vi "LEBITlib.deviceToLoad.vi"(1 "DeviceName":string) -> (0 "DeviceIsToLoad":bool)   [LabVIEW 2014, in "LEBITLib.lvlib"]
doc: "Checks, if a device object must be instantiated. The following convention is used.\n\nIf the object name starts with a \"*\", the device object is ignored and will not be used"
uses:
  LEBITLib.lvlib
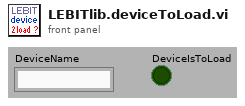
[diagram p1: front panel]
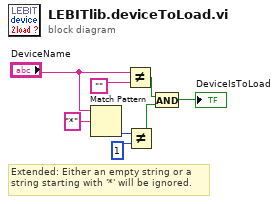
[diagram p0: block diagram]
diagram:
  # "Extended: Either an empty string or a\nstring starting with '*' will be ignored."
  n1 = Match Pattern(string="DeviceName", regular expression="*") -> (offset past match=w7:i32)  [unwired: 1 in, 3 out]
  n2 = Not Equal?(x="DeviceName", y="") -> (x != y?=w4:bool)
  n3 = Not Equal?(x=w7, y=1) -> (x != y?=w3:bool)
  n4 = And(x=w4, y=w3) -> (x .and. y?=→"DeviceIsToLoad":bool)
